vi "XCTL_Background_Service.vi"() -> ()   [LabVIEW 2012, in "WaveGraphX.xctl"]
doc: "此VI为后台程序, 持续运行, 为图例的移动服务.\nVI执行属性为可重入, 为每个对象创建副本."
uses:
  WaveGraphX.xctl
  <vilib>/Utility/miscctls.llb/LVPoint32TypeDef.ctl
panel:
  in  "峰值图例拖动坐标 队列":refnum<queue>
  in  "统计图例拖动坐标 队列":refnum<queue>
  in  "控件引用簇 队列":refnum<queue>
  in  "停止按钮":bool
  in  "曲线图例队列引用":refnum<queue>
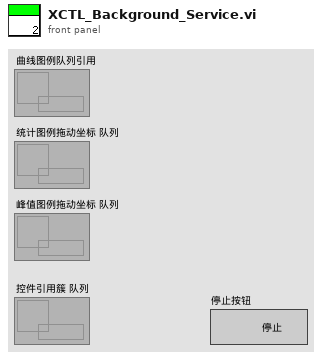
[diagram p1: front panel]
types:
  T1 = cluster{"图例拖动State":refnum<vi>, "统计图例拖动State":refnum<vi>, "峰值图例拖动State":refnum<vi>, "图例":refnum<vi>, "统计图例":refnum<vi>, "峰值图例":refnum<vi>}
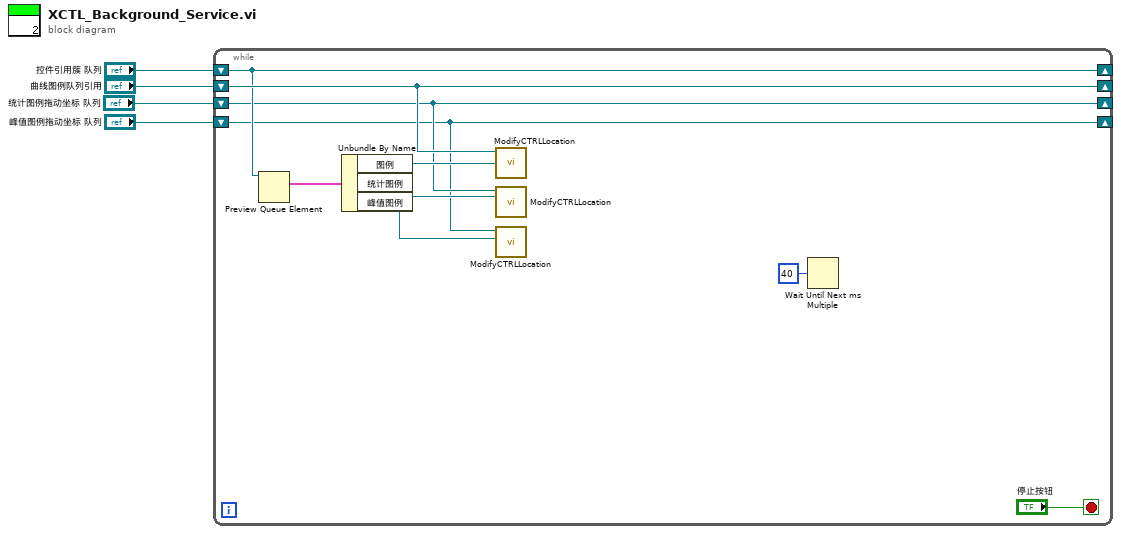
[diagram p0: block diagram]
diagram:
  n1 = while {
    shift-right: [w14] -> _
    shift-left: "曲线图例队列引用" -> [w14]
    shift-right: [w12] -> _
    shift-left: "控件引用簇 队列" -> [w12]
    shift-right: [w9] -> _
    shift-left: "统计图例拖动坐标 队列" -> [w9]
    shift-right: [w6] -> _
    shift-left: "峰值图例拖动坐标 队列" -> [w6]
    stop <- "停止按钮" stop-if-true
    n2 = Preview Queue Element(queue=w12) -> (element=w11:T1)  [unwired: 2 in, 3 out]
    n3 = Unbundle By Name(w11) -> ("图例"=w10:refnum<vi>, "统计图例"=w8:refnum<vi>, "峰值图例"=w7:refnum<vi>)
    n4 = call "ModifyCTRLLocation.vi"("图例"=w10, "队列输入"=w14) -> ()  [unwired: 10 in]
    n5 = call "ModifyCTRLLocation.vi"("图例"=w8, "队列输入"=w9) -> ()  [unwired: 10 in]
    n6 = call "ModifyCTRLLocation.vi"("图例"=w7, "队列输入"=w6) -> ()  [unwired: 10 in]
    n7 = Wait Until Next ms Multiple(millisecond multiple=u32 40 ("毫秒倍数")) -> ()  [unwired: 1 out]
  }
